vi "Init Nest Controls.vi"(8 "error in (no error)":errorcluster, 11 "Nest Cluster":refnum<vi>) -> (0 "error out":errorcluster)   [LabVIEW 2015]
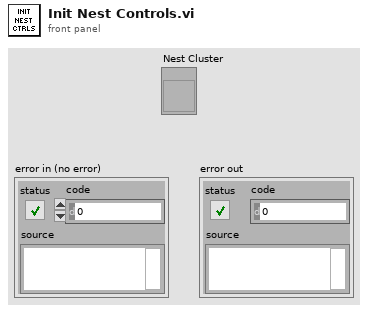
[diagram p1: front panel]
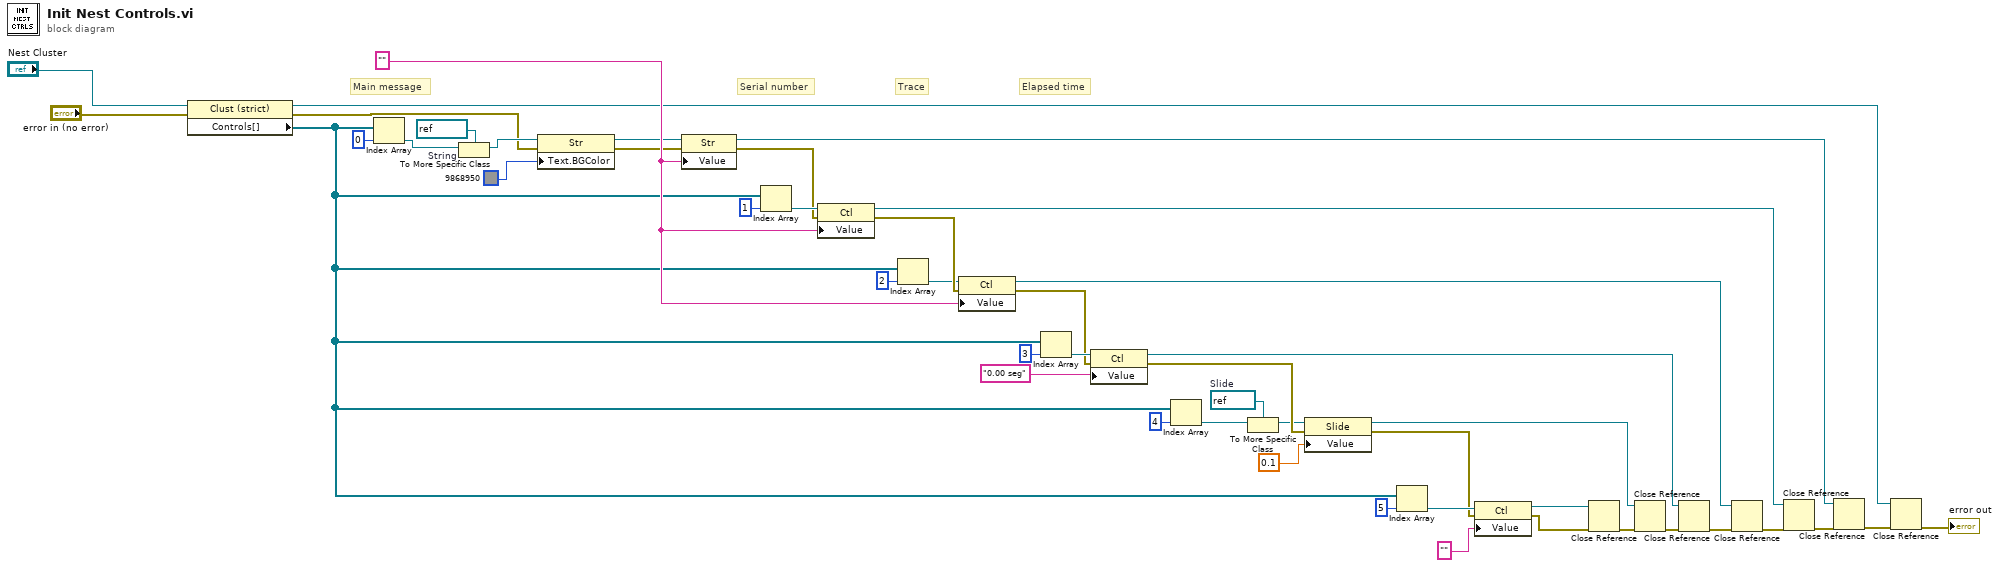
[diagram p0: block diagram]
diagram:
  w13 = refnum<vi> refnum  # Slide
  w23 = refnum<vi> refnum  # String
  w39 = ""
  # "Elapsed time"
  # "Trace"
  # "Serial number"
  # "Main message"
  n1 = property class="Clust (strict)"(reference="Nest Cluster", error in="error in (no error)") -> (reference out=w27:refnum<vi>, error out=w20:errorcluster, "Controls[]"=w8:refnum<vi>[])
  n2 = Index Array(array=w8, index=0) -> (element=w24:refnum<vi>)
  n3 = To More Specific Class(target class=w23, reference=w24) -> (specific class reference=w22:refnum<vi>)  [unwired: 1 in, 1 out]
  n4 = property class="Str"(reference=w22, error in=w20, "Text.BGColor"=u32 9868950) -> (reference out=w25:refnum<vi>, error out=w19:errorcluster)
  n5 = property class="Str"(reference=w25, error in=w19, "Value"=w39) -> (reference out=w29:refnum<vi>, error out=w43:errorcluster)
  n6 = Index Array(array=w8, index=1) -> (element=w44:refnum<vi>)
  n7 = property class="Ctl"(reference=w44, error in=w43, "Value"=w39) -> (reference out=w30:refnum<vi>, error out=w41:errorcluster)
  n8 = Index Array(array=w8, index=2) -> (element=w40:refnum<vi>)
  n9 = property class="Ctl"(reference=w40, error in=w41, "Value"=w39) -> (reference out=w31:refnum<vi>, error out=w36:errorcluster)
  n10 = Index Array(array=w8, index=3) -> (element=w37:refnum<vi>)
  n11 = property class="Ctl"(reference=w37, error in=w36, "Value"="0.00 seg") -> (reference out=w16:refnum<vi>, error out=w15:errorcluster)
  n12 = Index Array(array=w8, index=4) -> (element=w14:refnum<vi>)
  n13 = To More Specific Class(target class=w13, reference=w14) -> (specific class reference=w12:refnum<vi>)  [unwired: 1 in, 1 out]
  n14 = property class="Slide"(reference=w12, error in=w15, "Value"=0.1) -> (reference out=w1:refnum<vi>, error out=w2:errorcluster)
  n15 = Index Array(array=w8, index=5) -> (element=w7:refnum<vi>)
  n16 = property class="Ctl"(reference=w7, error in=w2, "Value"="") -> (reference out=w4:refnum<vi>, error out=w3:errorcluster)
  n17 = Close Reference(reference=w4, error in (no error)=w3) -> (error out=w5:errorcluster)
  n18 = Close Reference(reference=w1, error in (no error)=w5) -> (error out=w17:errorcluster)
  n19 = Close Reference(reference=w16, error in (no error)=w17) -> (error out=w34:errorcluster)
  n20 = Close Reference(reference=w31, error in (no error)=w34) -> (error out=w33:errorcluster)
  n21 = Close Reference(reference=w30, error in (no error)=w33) -> (error out=w32:errorcluster)
  n22 = Close Reference(reference=w29, error in (no error)=w32) -> (error out=w28:errorcluster)
  n23 = Close Reference(reference=w27, error in (no error)=w28) -> (error out=→"error out":errorcluster)
